vi "Keithley 24XX DCV Source Config.vi"(0 "VISA resource name":refnum<visa-resource-name>, 1 "Mode Selection (Fixed:0)":enum16{"Fixed", "Sweep", "List"}(ring), 3 "Range (Default:0)":T1(ring), 4 "Range Value (Volts)":dbl min=-1100.0 max=1100.0 step=5e-06 format="%.6e", 5 "List Requirement":bool, 7 "error in":T2, 8 "Sweep Parameters to Use":bool, 9 "List of Values (Up to 100, separated by commas)":string, 12 "Start Value":dbl min=-1100.0 max=1100.0 step=5e-06 format="%.6e", 13 "Stop Value":dbl min=-1100.0 max=1100.0 step=5e-06 format="%.6e", 14 "Center Value":dbl min=-1100.0 max=1100.0 step=5e-06 format="%.6e", 15 "Span Value":dbl min=-1100.0 max=1100.0 step=5e-06 format="%.11e", 16 "Sweep Direction/Sweep Spacing":u16(ring) items=["Sweep Up / Linear Spacing", "Sweep Down / Linear Spacing", "Sweep Up / Log Spacing", "Sweep Down / Log Spacing"], 17 "Step Value/Points":dbl min=-1100.0 max=2500.0 step=5e-06 format="%.6e", 18 "Output Mode":bool, 21 "Level (Default:0)":u16(ring) items=["Default 0V", "Minimum", "Maximum", "By Value"], 23 "Output Value (Volts)":dbl min=-1100.0 max=1100.0 step=5e-06 format="%.6e", 24 "Triggered Level (Default:0)":u16(ring) items=["Default 0V", "Minimum", "Maximum", "By Value"], 25 "Triggered Value (Volts)":dbl min=-1100.0 max=1100.0 step=5e-06 format="%.6e") -> (20 "dup VISA Session":refnum<visa-resource-name>, 27 "error out":T2)   [LabVIEW 2024]
doc: "This VI is used to configure the settings for DC Volts Sourcing. \n\nParameters:\nGPIB Address: Default to 24\n\nMode Selection:\n0 = Fixed (Default)\n1 = Sweep\n2 = List\n\nRange:\n0 = Default 20V Range (Default)\n1 = Minimum Range\n2 = Maximum Range\n3 = Set Range by value\n4 = Autorange on\n5 = Autorange off\n\nRange Value: -1100 TO +1100, 5uV steps\n\nFixed Level Current Source Parameters:\nOutput Mode:\nTRUE = Triggered\nFALSE = Immediate (Default)\n\nLevel:\n0 = 0V (Default)\n1 = Minimum\n2 = Maximum\n3 = Set by value\n\nOutput Value: -1100 TO +1100, 5uV steps\n\nTriggered Level:\n0 = 0V (Default)\n1 = Minimum\n2 = Maximum\n3 = Set by value\n\nTriggered Value: -1100 TO +1100, 5uV steps\n\nSweep Current Source Parameters:\nSweep Parameters to Use:\nFALSE = Start/Stop (Default)\nTRUE = Center Span\n\nStart Value: = -1100 TO +1100, 5uV steps\nStop Value: = -1100 TO +1100, 5uV steps\nCenter Value: = -1100 TO +1100, 5uV steps\nSpan Value: = -1100 TO +1100, 5uV steps\n\nSweep Direction / Sweep Spacing\n0 = Sweep Up / Linear Spacing (Default)\n1 = Sweep Down / Linear Spacing\n2 = Sweep Up / Log Spacing\n3 = Sweep Down / Log Spacing\n\nStep Value/Points: -1100 to 2500\nNOTE: For Linear sweeps, the value takes on the STEP value from -1100 to +1100. For Logarithmic sweeps, POINTS value is used with a range from 1 to 2500. Please make sure that you use the correct value for the proper sweep.\n\nCurrent List Source Parameters\nList Requirement:\nFALSE = Create (Default)\nTRUE = Append\n\nList of Values: Defines a list of source values up to 100 for the list sourcing mode. Example: 1.0, 2.0, 3.0\nCommas MUST separate the values. A list of up to 2500 points can be made by appending multiple lists.\n\nCalculation to keep in mind:\nCENTER = (START + STOP) /2\nSPAN = STOP -START\nSTART = CENTER - (SPAN/2)\nSTOP = CENTER + (SPAN/2)\nPOINTS = [(STOP - START) / STEP] +1\nPOINTS = (SPAN / STEP) +1"
panel:
  # "Fixed Level Voltage Source Parameters"
  # "Triggered\nImmediate"
  # "Sweep Voltage Source Parameters"
  # "Voltage List Source Parameters"
  # "Center/Span\nStart/Stop"
  # "Append\nCreate"
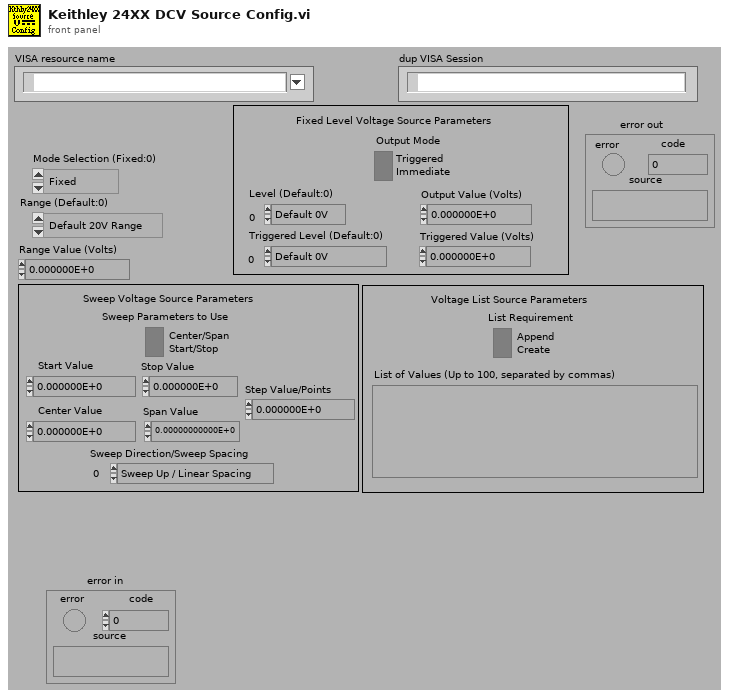
[diagram p1: front panel]
types:
  T1 = enum16{"Default 20V Range", "Minimum", "Maximum", "By Value", "Auto On", "Auto Off"}
  T2 = cluster{"error":bool, "code":i32, "source":string}
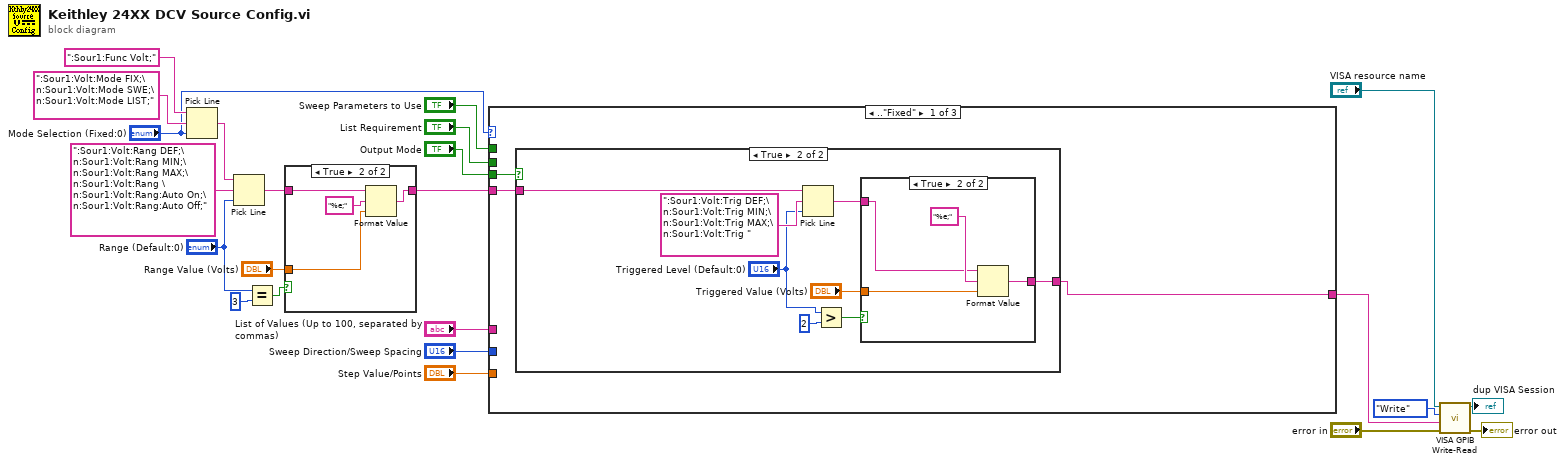
[diagram p0: block diagram]
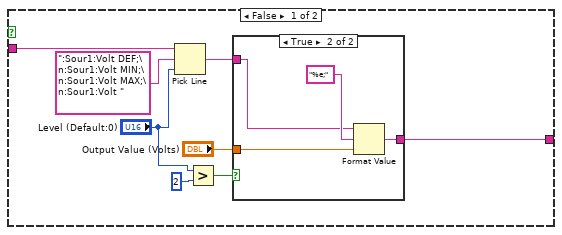
[diagram p3: hidden frame]
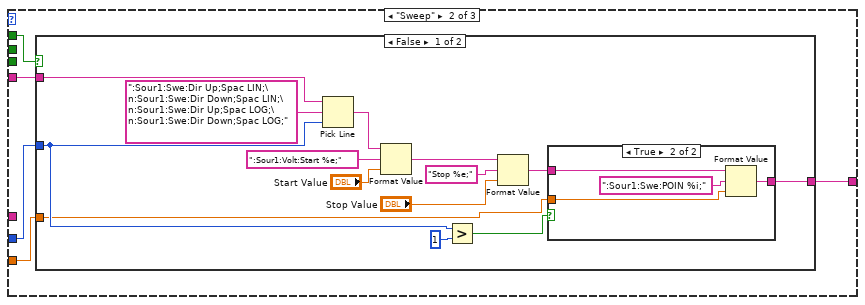
[diagram p6: hidden frame]
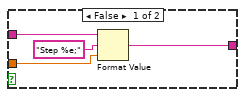
[diagram p7: hidden frame]
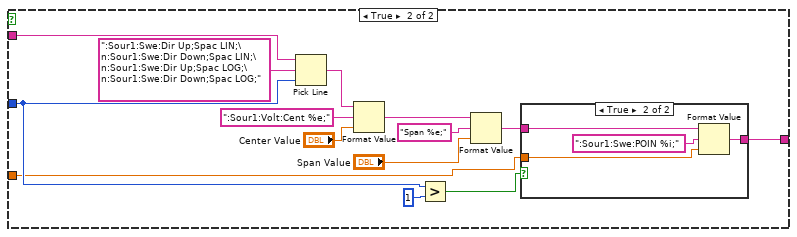
[diagram p8: hidden frame]
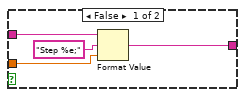
[diagram p9: hidden frame]
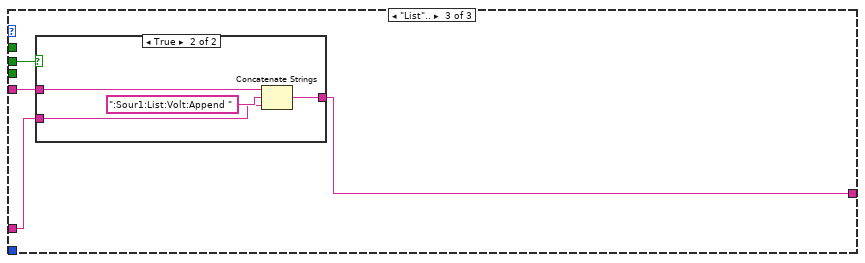
[diagram p10: hidden frame]
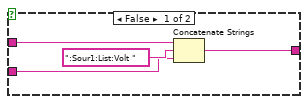
[diagram p11: hidden frame]
diagram:
  n1 = Pick Line(string ("")=":Sour1:Func Volt;", multi-line string=":Sour1:Volt:Mode FIX;\n:Sour1:Volt:Mode SWE;\n:Sour1:Volt:Mode LIST;", line index="Mode Selection (Fixed:0)") -> (output string=w17:string)
  n2 = Pick Line(string ("")=w17, multi-line string=":Sour1:Volt:Rang DEF;\n:Sour1:Volt:Rang MIN;\n:Sour1:Volt:Rang MAX;\n:Sour1:Volt:Rang \n:Sour1:Volt:Rang:Auto On;\n:Sour1:Volt:Rang:Auto Off;", line index="Range (Default:0)") -> (output string=w19:string)
  n3 = Equal?(x="Range (Default:0)", y=3) -> (x = y?=w13:bool)
  n4 = case shown="True" w13 {
    tunnel: [w24 w27] -> w15
    tunnel: w19 -> [w24 w26]
    tunnel: "Range Value (Volts)" -> [_ w25]
    frame False {
    }
    frame True {
      n5 = Format Value(string ("")=w26, format string="%e;", value (0)=w25) -> (output string=w27:string)
    }
  }
  n6 = case shown="..\"Fixed\"" "Mode Selection (Fixed:0)" {
    tunnel: "Output Mode" -> [w31 _ _]
    tunnel: w15 -> [w30 w62 w109]
    tunnel: "Step Value/Points" -> [_ w61 _]
    tunnel: [w29 w58 w107] -> w3
    tunnel: "List Requirement" -> [_ _ w110]
    tunnel: "List of Values (Up to 100, separated by commas)" -> [_ _ w108]
    tunnel: "Sweep Direction/Sweep Spacing" -> [_ w60 _]
    tunnel: "Sweep Parameters to Use" -> [_ w59 _]
    frame .."Fixed" {
      n7 = case shown="True" w31 {
        tunnel: [w33 w47] -> w29
        tunnel: w30 -> [w32 w45]
        frame False {
          n8 = Pick Line(string ("")=w32, multi-line string=":Sour1:Volt DEF;\n:Sour1:Volt MIN;\n:Sour1:Volt MAX;\n:Sour1:Volt ", line index="Level (Default:0)") -> (output string=w34:string)
          n9 = Greater?(x="Level (Default:0)", y=2) -> (0:w36:bool)
          n10 = case shown="True" w36 {
            tunnel: "Output Value (Volts)" -> [_ w43]
            tunnel: [w40 w42] -> w33
            tunnel: w34 -> [w40 w41]
            frame False {
            }
            frame True {
              n11 = Format Value(string ("")=w41, format string="%e;", value (0)=w43) -> (output string=w42:string)
            }
          }
        }
        frame True {
          n12 = Pick Line(string ("")=w45, multi-line string=":Sour1:Volt:Trig DEF;\n:Sour1:Volt:Trig MIN;\n:Sour1:Volt:Trig MAX;\n:Sour1:Volt:Trig ", line index="Triggered Level (Default:0)") -> (output string=w49:string)
          n13 = Greater?(x="Triggered Level (Default:0)", y=2) -> (0:w51:bool)
          n14 = case shown="True" w51 {
            tunnel: [w53 w56] -> w47
            tunnel: w49 -> [w53 w55]
            tunnel: "Triggered Value (Volts)" -> [_ w54]
            frame False {
            }
            frame True {
              n15 = Format Value(string ("")=w55, format string="%e;", value (0)=w54) -> (output string=w56:string)
            }
          }
        }
      }
    }
    frame "Sweep" {
      n16 = case shown="False" w59 {
        tunnel: w62 -> [w70 w92]
        tunnel: w61 -> [w65 w86]
        tunnel: w60 -> [w69 w91]
        tunnel: [w63 w85] -> w58
        frame False {
          n17 = Pick Line(string ("")=w70, multi-line string=":Sour1:Swe:Dir Up;Spac LIN;\n:Sour1:Swe:Dir Down;Spac LIN;\n:Sour1:Swe:Dir Up;Spac LOG;\n:Sour1:Swe:Dir Down;Spac LOG;", line index=w69) -> (output string=w68:string)
          n18 = Format Value(string ("")=w68, format string=":Sour1:Volt:Start %e;", value (0)="Start Value") -> (output string=w76:string)
          n19 = Greater?(x=w69, y=1) -> (0:w66:bool)
          n20 = Format Value(string ("")=w76, format string="Stop %e;", value (0)="Stop Value") -> (output string=w67:string)
          n21 = case shown="True" w66 {
            tunnel: [w79 w83] -> w63
            tunnel: w67 -> [w78 w82]
            tunnel: w65 -> [w77 w81]
            frame False {
              n22 = Format Value(string ("")=w78, format string="Step %e;", value (0)=w77) -> (output string=w79:string)
            }
            frame True {
              n23 = Format Value(string ("")=w82, format string=":Sour1:Swe:POIN %i;", value (0)=w81) -> (output string=w83:string)
            }
          }
        }
        frame True {
          n24 = Pick Line(string ("")=w92, multi-line string=":Sour1:Swe:Dir Up;Spac LIN;\n:Sour1:Swe:Dir Down;Spac LIN;\n:Sour1:Swe:Dir Up;Spac LOG;\n:Sour1:Swe:Dir Down;Spac LOG;", line index=w91) -> (output string=w89:string)
          n25 = Format Value(string ("")=w89, format string=":Sour1:Volt:Cent %e;", value (0)="Center Value") -> (output string=w98:string)
          n26 = Greater?(x=w91, y=1) -> (0:w88:bool)
          n27 = Format Value(string ("")=w98, format string="Span %e;", value (0)="Span Value") -> (output string=w87:string)
          n28 = case shown="True" w88 {
            tunnel: w87 -> [w99 w103]
            tunnel: w86 -> [w101 w106]
            tunnel: [w100 w104] -> w85
            frame False {
              n29 = Format Value(string ("")=w99, format string="Step %e;", value (0)=w101) -> (output string=w100:string)
            }
            frame True {
              n30 = Format Value(string ("")=w103, format string=":Sour1:Swe:POIN %i;", value (0)=w106) -> (output string=w104:string)
            }
          }
        }
      }
    }
    frame "List".. {
      n31 = case shown="True" w110 {
        tunnel: w109 -> [w114 w117]
        tunnel: w108 -> [w112 w116]
        tunnel: [w111 w115] -> w107
        frame False {
          n32 = Concatenate Strings(w114, ":Sour1:List:Volt ", w112) -> (w111:string)
        }
        frame True {
          n33 = Concatenate Strings(w117, ":Sour1:List:Volt:Append ", w116) -> (w115:string)
        }
      }
    }
  }
  n34 = call "VISA GPIB Write-Read.vi"("error in (no error)"="error in", "Command"=w3, "Action"=enum16{"Write", "Read", "Write & Read"}."Write", "VISA resource name"="VISA resource name") -> ("error out"=→"error out":errorcluster, "dup VISA Session"=→"dup VISA Session":refnum<visa-resource-name>)  [unwired: 4 in, 2 out]
